vi "CRYMR_Margin.vi"(2 "To":cluster{dbl, dbl}[](array[cluster]) {"?" format="%.2f"; "?" format="%.2f"}, 3 "From":cluster{dbl, dbl}[](array[cluster]) {"?" format="%.2f"; "?" format="%.2f"}, 4 "Direction":enum16{"Upwards", "Downwards"}(ring)) -> (0 "X":dbl=-inf format="%.2f", 1 "Margin":dbl=inf format="%.2p")   [LabVIEW 2013]
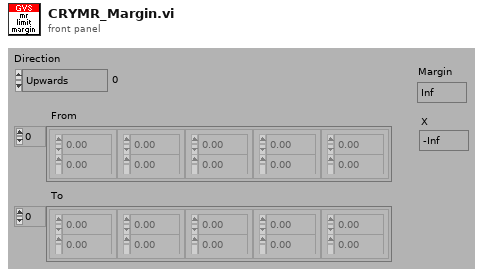
[diagram p1: front panel]
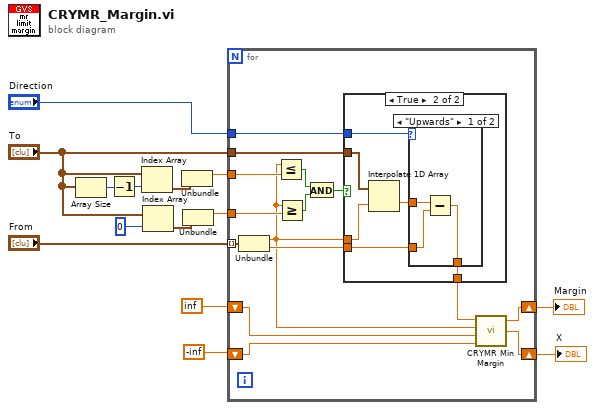
[diagram p0: block diagram]
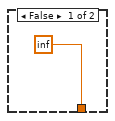
[diagram p2: hidden frame]
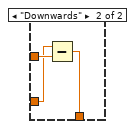
[diagram p3: hidden frame]
diagram:
  n1 = Array Size(array="To") -> (size(s)=w12:i32)
  n2 = Decrement(x=w12) -> (x-1=w11:i32)
  n3 = Index Array(array="To", index=w11) -> (element=w14:cluster{dbl, dbl})
  n4 = Index Array(array="To", index=0) -> (element=w13:cluster{dbl, dbl})
  n5 = Unbundle(w14) -> (w8:dbl)  [unwired: 1 out]
  n6 = Unbundle(w13) -> (w9:dbl)  [unwired: 1 out]
  n7 = for {
    tunnel: w9 -> [w25]
    tunnel: "From" -> [w29] mode=indexing
    tunnel: "To" -> [w28]
    tunnel: w8 -> [w24]
    tunnel: "Direction" -> [w27]
    shift-right: [w20] -> w6
    shift-left: inf -> [w16]
    shift-right: [w15] -> w5
    shift-left: -inf -> [w19]
    n8 = Unbundle(w29) -> (w17:dbl, w26:dbl)
    n9 = Less Or Equal?(x=w17, y=w24) -> (x <= y?=w23:bool)
    n10 = Greater Or Equal?(x=w17, y=w25) -> (x >= y?=w22:bool)
    n11 = And(x=w23, y=w22) -> (x .and. y?=w21:bool)
    n12 = case shown="True" w21 {
      tunnel: w28 -> [_ w36]
      tunnel: w17 -> [_ w35]
      tunnel: w27 -> [_ w34]
      tunnel: w26 -> [_ w32]
      tunnel: [inf w31] -> w18
      frame False {
      }
      frame True {
        n13 = Interpolate 1D Array(1:w35, 2:w36) -> (0:w33:dbl)
        n14 = case shown="\"Upwards\"" w34 {
          tunnel: w33 -> [w39 w41]
          tunnel: w32 -> [w38 w40]
          tunnel: [w37 w42] -> w31
          frame "Upwards" {
            n15 = Subtract(x=w39, y=w38) -> (x-y=w37:dbl)
          }
          frame "Downwards" {
            n16 = Subtract(x=w40, y=w41) -> (x-y=w42:dbl)
          }
        }
      }
    }
    n17 = call "CRYMR Min Margin.vi"("Lower X"=w19, "Lower Margin"=w16, "Upper X"=w17, "Upper Margin"=w18) -> ("X"=w15:dbl, "Min Margin"=w20:dbl)  [unwired: 1 out]
  }
  "Margin" <- w6
  "X" <- w5
